vi "Plan Path.vi"(8 "error in (no error)":errorcluster, 10 "Controle":T1, 11 "map reference in":refnum<data-value>) -> (0 "error out":errorcluster, 2 "Indicator":T1, 3 "map reference out":refnum<data-value>)   [LabVIEW 2011]
uses:
  <vilib>/robotics/Navigation/shared/WorldMap/OccupancyGridWorldMap/NI_Robotics_OccupancyGridWorldMap.lvclass
  <vilib>/robotics/Navigation/NI_Robotics_Navigation .lvlib
panel:
  out "appended array":dbl[](array[numeric])
  out "intensity values":dbl[][](array[numeric])
  out "goal node":cluster{"X":i32, "Y":i32}={"X"=32, "Y"=32}
  out "start node":cluster{"X":i32, "Y":i32}={"X"=3, "Y"=3}
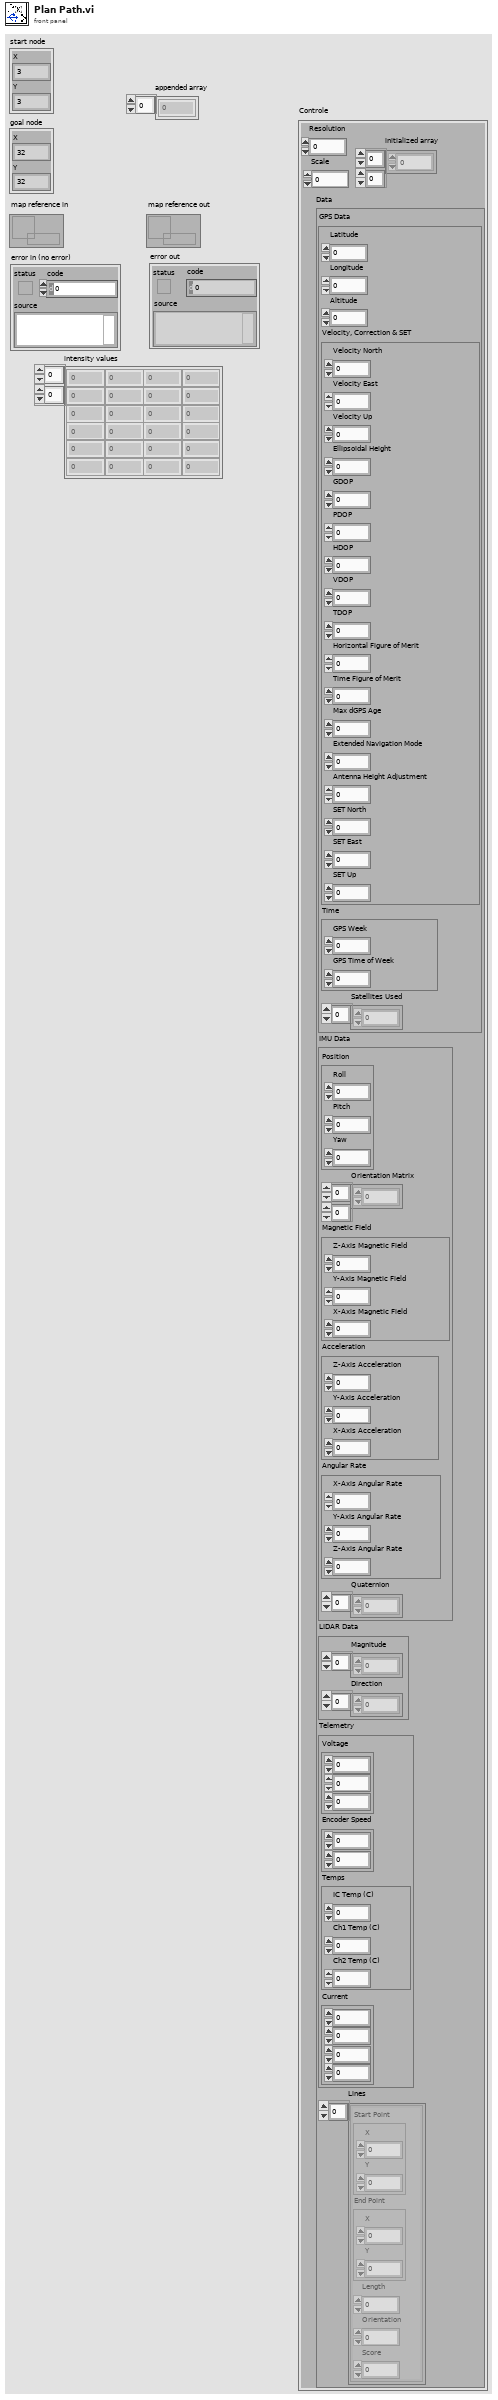
[diagram p1: front panel]
types:
  T1 = cluster{"Resolution":i32, "Scale":dbl, "Data":cluster{"GPS Data":cluster{"Latitude":dbl, "Longitude":dbl, "Altitude":dbl, "Velocity, Correction & SET":cluster{"Velocity North":dbl, "Velocity East":dbl, "Velocity Up":dbl, "Ellipsoidal Height":dbl, "GDOP":sgl, "PDOP":sgl, "HDOP":sgl, "VDOP":sgl, "TDOP":sgl, "Horizontal Figure of Merit":u8, "Time Figure of Merit":u8, "Max dGPS Age":sgl, "Extended Navigation Mode":u8, "Antenna Height Adjustment ":dbl, "SET North":i32, "SET East":i32, "SET Up":i32}, "Time":cluster{"GPS Week":u16, "GPS Time of Week":sgl}, "Satellites Used":i32[]}, "IMU Data":cluster{"Position":cluster{"Roll":dbl, "Pitch":dbl, "Yaw":dbl}, "Orientation Matrix":dbl[][], "Magnetic Field":cluster{"Z-Axis Magnetic Field":dbl, "Y-Axis Magnetic Field":dbl, "X-Axis Magnetic Field":dbl}, "Acceleration":cluster{"Z-Axis Acceleration":dbl, "Y-Axis Acceleration":dbl, "X-Axis Acceleration":dbl}, "Angular Rate":cluster{"X-Axis Angular Rate":dbl, "Y-Axis Angular Rate":dbl, "Z-Axis Angular Rate":dbl}, "Quaternion":dbl[]}, "LIDAR Data":cluster{"Magnitude":dbl[], "Direction":dbl[]}, "Telemetry":cluster{"Voltage":cluster{sgl, sgl, sgl}, "Encoder Speed":cluster{i32, i32}, "Temps":cluster{"IC Temp (C)":i32, "Ch1 Temp (C)":i32, "Ch2 Temp (C)":i32}, "Current":cluster{dbl, dbl, dbl, dbl}}, "Lines":cluster{"Start Point":cluster{"X":sgl, "Y":sgl}, "End Point":cluster{"X":sgl, "Y":sgl}, "Length":dbl, "Orientation":dbl, "Score":dbl}[]}, "initialized array":dbl[][]}
  T2 = cluster{"Latitude":dbl, "Longitude":dbl, "Altitude":dbl, "Velocity, Correction & SET":cluster{"Velocity North":dbl, "Velocity East":dbl, "Velocity Up":dbl, "Ellipsoidal Height":dbl, "GDOP":sgl, "PDOP":sgl, "HDOP":sgl, "VDOP":sgl, "TDOP":sgl, "Horizontal Figure of Merit":u8, "Time Figure of Merit":u8, "Max dGPS Age":sgl, "Extended Navigation Mode":u8, "Antenna Height Adjustment ":dbl, "SET North":i32, "SET East":i32, "SET Up":i32}, "Time":cluster{"GPS Week":u16, "GPS Time of Week":sgl}, "Satellites Used":i32[]}
  T3 = cluster{"Position":cluster{"Roll":dbl, "Pitch":dbl, "Yaw":dbl}, "Orientation Matrix":dbl[][], "Magnetic Field":cluster{"Z-Axis Magnetic Field":dbl, "Y-Axis Magnetic Field":dbl, "X-Axis Magnetic Field":dbl}, "Acceleration":cluster{"Z-Axis Acceleration":dbl, "Y-Axis Acceleration":dbl, "X-Axis Acceleration":dbl}, "Angular Rate":cluster{"X-Axis Angular Rate":dbl, "Y-Axis Angular Rate":dbl, "Z-Axis Angular Rate":dbl}, "Quaternion":dbl[]}
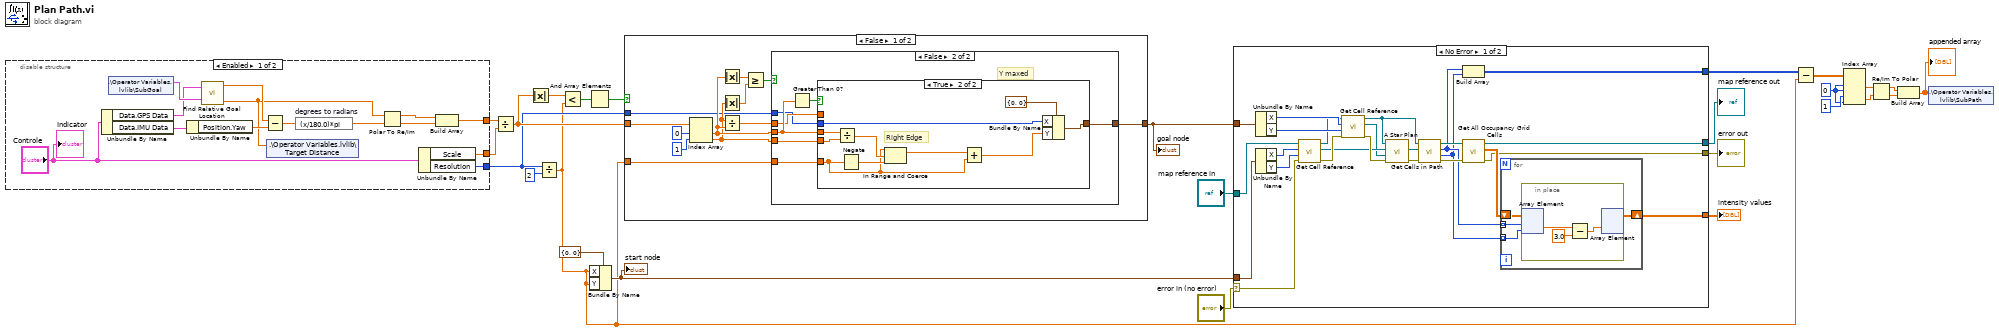
[diagram p0: block diagram]
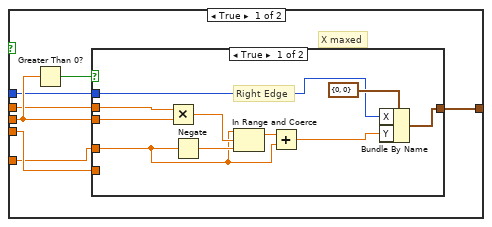
[diagram p3: hidden frame]
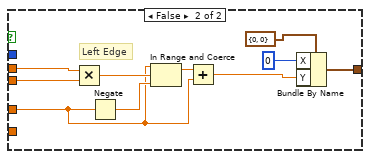
[diagram p4: hidden frame]
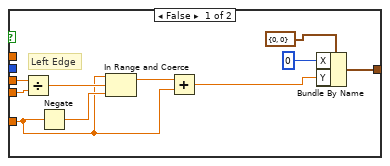
[diagram p5: hidden frame]
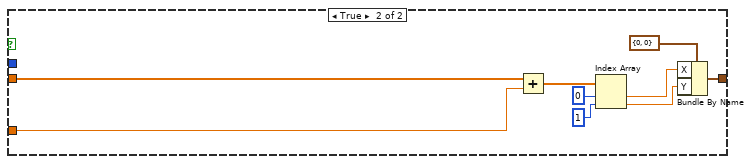
[diagram p6: hidden frame]
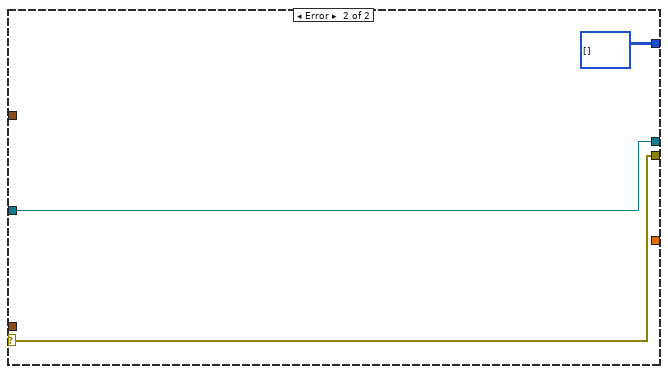
[diagram p7: hidden frame]
diagram:
  w14 = 0 ("index (row)")
  n1 = disable-structure shown="Enabled" {
    disable-tunnel: [w32 _] -> w2
    disable-tunnel: [w31 _] -> w3
    disable-tunnel: [w30 _] -> w4
    frame Enabled {
      n2 = Unbundle By Name("Controle") -> ("Data.GPS Data"=w29:T2, "Data.IMU Data"=w28:T3)
      n3 = shared-variable ".\\Operator Variables.lvlib\\SubGoal"() -> (w40:T2)  [unwired: 1 in, 1 out]
      n4 = Unbundle By Name(w28) -> ("Position.Yaw"=w38:dbl)
      n5 = call "Find Relative Goal Location.vi"("Current Position"=w29, "Goal Position"=w40) -> ("Target Heading (deg)"=w39:dbl, "Target Distance"=w36:dbl)  [unwired: 1 out]
      n6 = Subtract(x=w39, y=w38) -> (x-y=w37:dbl)
      n7 = shared-variable ".\\Operator Variables.lvlib\\Target Distance"(w36) -> ()  [unwired: 1 in, 1 out]
      n8 = expression code="(x/180.0)*pi" "degrees to radians"(w37) -> (w35:dbl)
      n9 = Polar To Re/Im(2:w35, 3:w36) -> (0:w33:dbl, 1:w34:dbl)
      n10 = Unbundle By Name("Controle") -> ("Scale"=w30:dbl, "Resolution"=w31:i32)
      n11 = Build Array(w34, w33) -> (w32:dbl[])
      "Indicator" <- "Controle"
    }
    frame Disabled {
    }
  }
  n12 = Divide(x=w2, y=w4) -> (x/y=w5:dbl[])
  n13 = Absolute Value(x=w5) -> (abs(x)=w6:dbl[])
  n14 = Divide(x=w3, y=2 ("value")) -> (x/y=w1:dbl)
  n15 = Less?(x=w6, y=w1) -> (x < y?=w20:bool[])
  n16 = And Array Elements(Boolean array=w20) -> (logical AND=w21:bool)
  n17 = Bundle By Name(cluster=cluster{"X":i32, "Y":i32} {"X"=0, "Y"=0} ("goal node"), "X"=w1, "Y"=w1) -> (w17:cluster{"X":i32, "Y":i32})
  "start node" <- w17
  n18 = case shown="False" w21 {
    tunnel: w5 -> [w43 w115]
    tunnel: [w44 w108] -> w19
    tunnel: w3 -> [w42 _]
    tunnel: w1 -> [w41 w107]
    frame False {
      n19 = Index Array(array=w43, index #1=0 ("index"), index #2=1 ("index")) -> (element #1=w47:dbl, element #2=w46:dbl)
      n20 = Absolute Value(x=w47) -> (abs(x)=w50:dbl)
      n21 = Absolute Value(x=w46) -> (abs(x)=w49:dbl)
      n22 = Divide(x=w46, y=w47) -> (x/y=w45:dbl)
      n23 = Greater Or Equal?(x=w50, y=w49) -> (x >= y?=w48:bool)
      n24 = case shown="False" w48 {
        tunnel: w47 -> [w57 w84]
        tunnel: w46 -> [w56 w83]
        tunnel: w45 -> [w55 w82]
        tunnel: [w58 w85] -> w44
        tunnel: w42 -> [w54 w81]
        tunnel: w41 -> [w53 w80]
        frame True {
          # "X maxed"
          n25 = Greater Than 0?(x=w57) -> (x > 0?=w59:bool)
          n26 = case shown="True" w59 {
            tunnel: [w68 w78] -> w58
            tunnel: w57 -> [w66 w76]
            tunnel: w56 -> [_ _]
            tunnel: w55 -> [w67 w77]
            tunnel: w54 -> [w63 _]
            tunnel: w53 -> [w60 w71]
            frame True {
              # "Right Edge"
              n27 = Multiply(x=w67, y=w66) -> (x*y=w65:dbl)
              n28 = Negate(x=w60) -> (-x=w61:dbl)
              n29 = In Range and Coerce(upper limit=w60, x=w65, lower limit=w61) -> (coerced(x)=w64:dbl)  [unwired: 1 out]
              n30 = Add(x=w64, y=w60) -> (x+y=w62:dbl)
              n31 = Bundle By Name(cluster=cluster{"X":i32, "Y":i32} {"X"=0, "Y"=0} ("goal node"), "X"=w63, "Y"=w62) -> (w68:cluster{"X":i32, "Y":i32})
            }
            frame False {
              # "Left Edge"
              n32 = Multiply(x=w77, y=w76) -> (x*y=w75:dbl)
              n33 = Negate(x=w71) -> (-x=w72:dbl)
              n34 = In Range and Coerce(upper limit=w71, x=w75, lower limit=w72) -> (coerced(x)=w74:dbl)  [unwired: 1 out]
              n35 = Add(x=w74, y=w71) -> (x+y=w73:dbl)
              n36 = Bundle By Name(cluster=cluster{"X":i32, "Y":i32} {"X"=0, "Y"=0} ("goal node"), "X"=0, "Y"=w73) -> (w78:cluster{"X":i32, "Y":i32})
            }
          }
        }
        frame False {
          # "Y maxed"
          n37 = Greater Than 0?(x=w84) -> (x > 0?=w86:bool)
          n38 = case shown="True" w86 {
            tunnel: [w95 w105] -> w85
            tunnel: w84 -> [w88 w99]
            tunnel: w83 -> [w87 w98]
            tunnel: w82 -> [_ _]
            tunnel: w81 -> [_ w97]
            tunnel: w80 -> [w90 w100]
            frame False {
              # "Left Edge"
              n39 = Divide(x=w88, y=w87) -> (x/y=w94:dbl)
              n40 = Negate(x=w90) -> (-x=w91:dbl)
              n41 = In Range and Coerce(upper limit=w90, x=w94, lower limit=w91) -> (coerced(x)=w93:dbl)  [unwired: 1 out]
              n42 = Add(x=w93, y=w90) -> (x+y=w92:dbl)
              n43 = Bundle By Name(cluster=cluster{"X":i32, "Y":i32} {"X"=0, "Y"=0} ("goal node"), "X"=0, "Y"=w92) -> (w95:cluster{"X":i32, "Y":i32})
            }
            frame True {
              # "Right Edge"
              n44 = Divide(x=w99, y=w98) -> (x/y=w104:dbl)
              n45 = Negate(x=w100) -> (-x=w101:dbl)
              n46 = In Range and Coerce(upper limit=w100, x=w104, lower limit=w101) -> (coerced(x)=w103:dbl)  [unwired: 1 out]
              n47 = Add(x=w103, y=w100) -> (x+y=w102:dbl)
              n48 = Bundle By Name(cluster=cluster{"X":i32, "Y":i32} {"X"=0, "Y"=0} ("goal node"), "X"=w97, "Y"=w102) -> (w105:cluster{"X":i32, "Y":i32})
            }
          }
        }
      }
    }
    frame True {
      n49 = Add(x=w115, y=w107) -> (x+y=w113:dbl[])
      n50 = Index Array(array=w113, index #1=0 ("index"), index #2=1 ("index")) -> (element #1=w110:dbl, element #2=w109:dbl)
      n51 = Bundle By Name(cluster=cluster{"X":i32, "Y":i32} {"X"=0, "Y"=0} ("goal node"), "X"=w110, "Y"=w109) -> (w108:cluster{"X":i32, "Y":i32})
    }
  }
  "goal node" <- w19
  n52 = case shown="No Error" "error in (no error)" {
    selector: "error in (no error)" -> [w124 w149]
    tunnel: "map reference in" -> [w125 w150]
    tunnel: w19 -> [w123 _]
    tunnel: w17 -> [w122 _]
    tunnel: [w121 _] -> w26
    tunnel: [w120 w150] -> w24
    tunnel: [w119 w149] -> w23
    tunnel: [w116 i32[][] []] -> w11
    frame No Error {
      n53 = Unbundle By Name(w123) -> ("X"=w139:i32, "Y"=w140:i32)
      n54 = Unbundle By Name(w122) -> ("X"=w137:i32, "Y"=w138:i32)
      n55 = call <vilib>:"Get Cell Reference.vi"("error in (no error)"=w124, "y"=w138, "x"=w137, "map reference in"=w125) -> ("error out"=w129:errorcluster, "cell reference"=w127:refnum<data-value>, "map reference out"=w133:refnum<data-value>)  [unwired: 4 in, 1 out]
      n56 = call <vilib>:"Get Cell Reference.vi"("error in (no error)"=w129, "y"=w140, "x"=w139, "map reference in"=w133) -> ("error out"=w134:errorcluster, "cell reference"=w126:refnum<data-value>, "map reference out"=w131:refnum<data-value>)  [unwired: 4 in, 1 out]
      n57 = call <vilib>:"A Star Plan.vi"("error in (no error)"=w134, "goal reference"=w126, "start reference"=w127, "map reference in"=w131) -> ("error out"=w135:errorcluster, "path references"=w132:refnum<data-value>[])  [unwired: 4 in, 2 out]
      n58 = call <vilib>:"Get Cells in Path.vi"("error in (no error)"=w135, "path references"=w132, "map reference in"=w131) -> ("error out"=w128:errorcluster, "y coordinates"=w117:i32[], "x coordinates"=w118:i32[], "map reference out"=w130:refnum<data-value>)  [unwired: 5 in]
      n59 = Build Array(w118, w117) -> (w116:i32[][])
      n60 = call <vilib>:"Get All Occupancy Grid Cells.vi"("error in (no error)"=w128, "map reference in"=w130) -> ("error out"=w119:errorcluster, "occupancy grid"=w136:dbl[][], "map reference out"=w120:refnum<data-value>)  [unwired: 7 in]
      n61 = for {
        tunnel: w117 -> [w142] mode=indexing
        tunnel: w118 -> [w143] mode=indexing
        shift-right: [w141] -> w121
        shift-left: w136 -> [w144]
        n62 = in-place {
          n63 = in-place-array #1(w144, w143, w142) -> (w146:dbl)
          n64 = Subtract(x=w146, y=3.0) -> (x-y=w145:dbl)
          n65 = in-place-array #1(w145) -> (w141:dbl[][])  [unwired: 2 out]
        }
      }
    }
    frame Error {
    }
  }
  "map reference out" <- w24
  "error out" <- w23
  "intensity values" <- w26
  n66 = Subtract(x=w11, y=w1) -> (x-y=w10:dbl[][])
  n67 = Index Array(array=w10, index (row) #1=w14, index (col) #1=w14, index (row) #2=1 ("index (row)"), index (col) #2=w14) -> (element #1=w13:dbl, element #2=w12:dbl)
  n68 = Re/Im To Polar(2:w12, 3:w13) -> (0:w8:dbl, 1:w9:dbl)
  n69 = Build Array(w9, w8) -> (w7:dbl[])
  "appended array" <- w7
  n70 = shared-variable ".\\Operator Variables.lvlib\\SubPath"(w7) -> ()  [unwired: 1 in, 1 out]
